vi "InitFromString.vi"(9 "ActionStack String":string) -> (1 "ActionStack out":refnum<class "Action.lvclass">[](array[class]))   [LabVIEW 2025]
doc: "Splits string via /n (new line)\nThen check for Args which can be passed in the JKI SM style (action >> arg)\nCan be followed by // for comments\nArgument encoding (case insensitive):\n<B>Bools</B>\nT/True\nF/False\n<B>Numerics</B>\nu8.. u64: numeric value\ni8.. i64: signed numeric value\ns.. d: floating point value\n<B>Special Strings</B>\nPath: File/Folder Path\n<B>Default</B>\nstring"
uses:
  Action.lvclass
  <vilib>/Utility/error.llb/Trim Whitespace One-Sided.vi
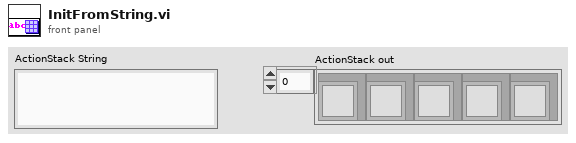
[diagram p1: front panel]
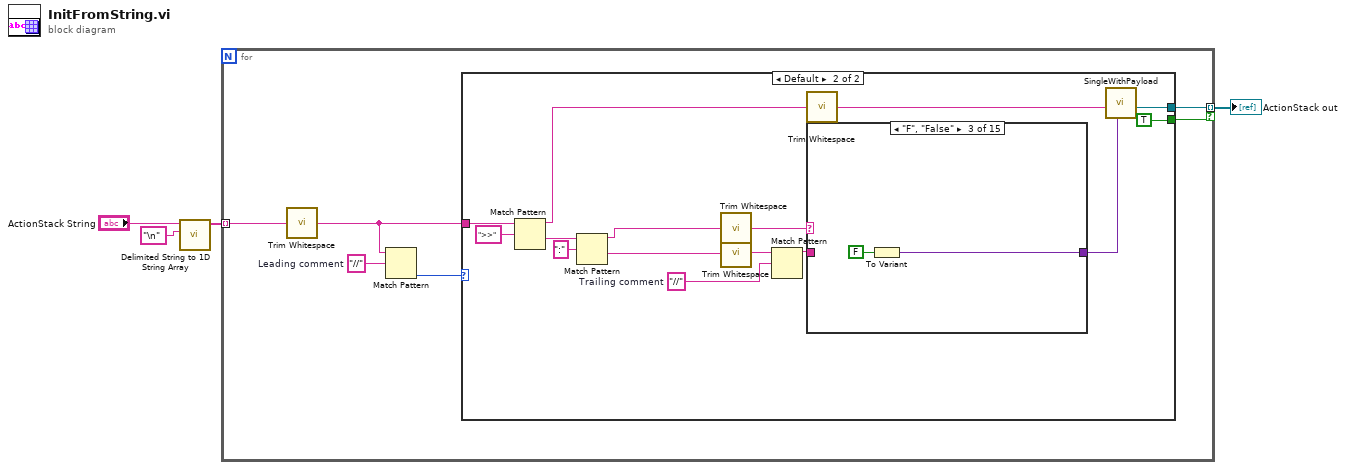
[diagram p0: block diagram]
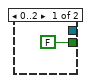
[diagram p2: hidden frame]
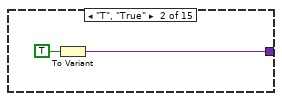
[diagram p4: hidden frame]
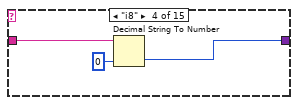
[diagram p5: hidden frame]
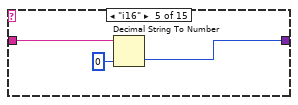
[diagram p6: hidden frame]
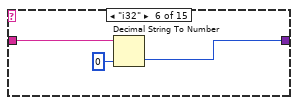
[diagram p7: hidden frame]
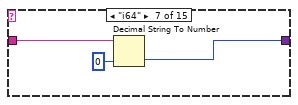
[diagram p8: hidden frame]
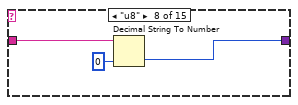
[diagram p9: hidden frame]
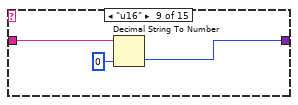
[diagram p10: hidden frame]
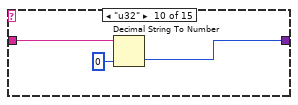
[diagram p11: hidden frame]
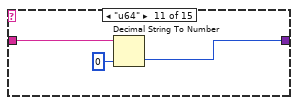
[diagram p12: hidden frame]
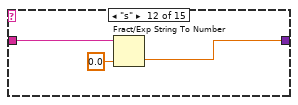
[diagram p13: hidden frame]
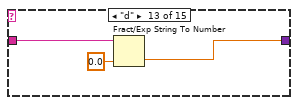
[diagram p14: hidden frame]
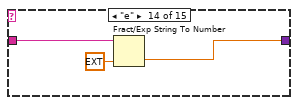
[diagram p15: hidden frame]
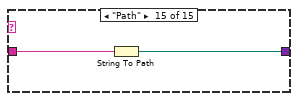
[diagram p16: hidden frame]
diagram:
  n1 = call <vilib>:"Delimited String to 1D String Array.vi"("delimiter"="\n", "delimited string"="ActionStack String") -> ("string array"=w2:string[])  [unwired: 9 in]
  n2 = for {
    tunnel: w2 -> [w8] mode=indexing
    tunnel: [w10] -> w1 mode=indexing if=w5
    w9 = "//"  # Leading comment
    n3 = call <vilib>:"Trim Whitespace.vi"("string"=w8) -> ("trimmed string"=w7:string)  [unwired: 1 in]
    n4 = Match Pattern(string=w7, regular expression=w9) -> (offset past match=w6:i32)  [unwired: 1 in, 3 out]
    n5 = case shown="Default" w6 {
      tunnel: [_ w12] -> w10
      tunnel: w7 -> [_ w16]
      tunnel: [FALSE TRUE] -> w5
      frame 0..2 {
      }
      frame Default {
        w17 = "//"  # Trailing comment
        n6 = Match Pattern(string=w16, regular expression=">>") -> (before substring=w25:string, after substring=w23:string)  [unwired: 1 in, 2 out]
        n7 = Match Pattern(string=w23, regular expression=":" ("search string/char (-)")) -> (before substring=w22:string, after substring=w21:string)  [unwired: 1 in, 2 out]
        n8 = call <vilib>:"Trim Whitespace.vi"("string"=w22) -> ("trimmed string"=w24:string)  [unwired: 1 in]
        n9 = call <vilib>:"Trim Whitespace.vi"("string"=w21) -> ("trimmed string"=w19:string)  [unwired: 1 in]
        n10 = Match Pattern(string=w19, regular expression=w17) -> (before substring=w18:string)  [unwired: 1 in, 3 out]
        n11 = call <vilib>:"Trim Whitespace.vi"("string"=w25) -> ("trimmed string"=w13:string)  [unwired: 1 in]
        n12 = case shown="\"F\", \"False\"" w24 {
          selector: w24 -> [w27 _ _ _ _ _ _ _ _ _ _ _ _ _ _]
          tunnel: [w27 w28 w30 w32 w35 w38 w41 w44 w47 w50 w53 w56 w59 w62 w65] -> w14
          tunnel: w18 -> [_ _ _ w34 w37 w40 w43 w46 w49 w52 w55 w58 w61 w64 w66]
          frame Default {
          }
          frame "T", "True" {
            n13 = To Variant(anything=TRUE) -> (Variant=w28:variant)
          }
          frame "F", "False" {
            n14 = To Variant(anything=FALSE) -> (Variant=w30:variant)
          }
          frame "i8" {
            n15 = Decimal String To Number(string=w34, default (0L)=i8 0 ("default (0 I32)")) -> (number=w32:i8)  [unwired: 1 in, 1 out]
          }
          frame "i16" {
            n16 = Decimal String To Number(string=w37, default (0L)=i16 0 ("default (0 I32)")) -> (number=w35:i16)  [unwired: 1 in, 1 out]
          }
          frame "i32" {
            n17 = Decimal String To Number(string=w40, default (0L)=0 ("default (0 I32)")) -> (number=w38:i32)  [unwired: 1 in, 1 out]
          }
          frame "i64" {
            n18 = Decimal String To Number(string=w43, default (0L)=i64 0 ("default (0 I32)")) -> (number=w41:i64)  [unwired: 1 in, 1 out]
          }
          frame "u8" {
            n19 = Decimal String To Number(string=w46, default (0L)=u8 0 ("default (0 I32)")) -> (number=w44:u8)  [unwired: 1 in, 1 out]
          }
          frame "u16" {
            n20 = Decimal String To Number(string=w49, default (0L)=u16 0 ("default (0 I32)")) -> (number=w47:u16)  [unwired: 1 in, 1 out]
          }
          frame "u32" {
            n21 = Decimal String To Number(string=w52, default (0L)=u32 0 ("default (0 I32)")) -> (number=w50:u32)  [unwired: 1 in, 1 out]
          }
          frame "u64" {
            n22 = Decimal String To Number(string=w55, default (0L)=u64 0 ("default (0 I32)")) -> (number=w53:u64)  [unwired: 1 in, 1 out]
          }
          frame "s" {
            n23 = Fract/Exp String To Number(string=w58, default (0 dbl)=sgl 0.0 ("default (0 I32)")) -> (number=w56:sgl)  [unwired: 2 in, 1 out]
          }
          frame "d" {
            n24 = Fract/Exp String To Number(string=w61, default (0 dbl)=0.0 ("default (0 I32)")) -> (number=w59:dbl)  [unwired: 2 in, 1 out]
          }
          frame "e" {
            n25 = Fract/Exp String To Number(string=w64, default (0 dbl)=ext 0.0 ("default (0 I32)")) -> (number=w62:ext)  [unwired: 2 in, 1 out]
          }
          frame "Path" {
            n26 = String To Path(string=w66) -> (path=w65:path)
          }
        }
        n27 = call "SingleWithPayload.vi"("Payload"=w14, "Action"=w13) -> ("ActionStack out"=w12:refnum<class "Action.lvclass">)  [unwired: 9 in]
      }
    }
  }
  "ActionStack out" <- w1
